vi "Read.vi"(8 "error in (no error)":errorcluster, 11 "Configuration Database API in":refnum<class "Configuration Database API.lvclass">) -> (0 "error out":errorcluster, 3 "Configuration Database API out":refnum<class "Configuration Database API.lvclass">)   [LabVIEW 2012, in "Configuration Database API.lvlib" / "Configuration Database API.lvclass"]
uses:
  Configuration Database API.lvclass
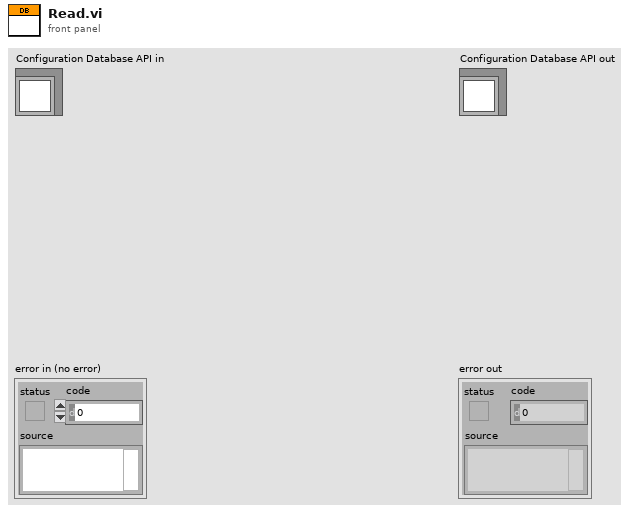
[diagram p1: front panel]
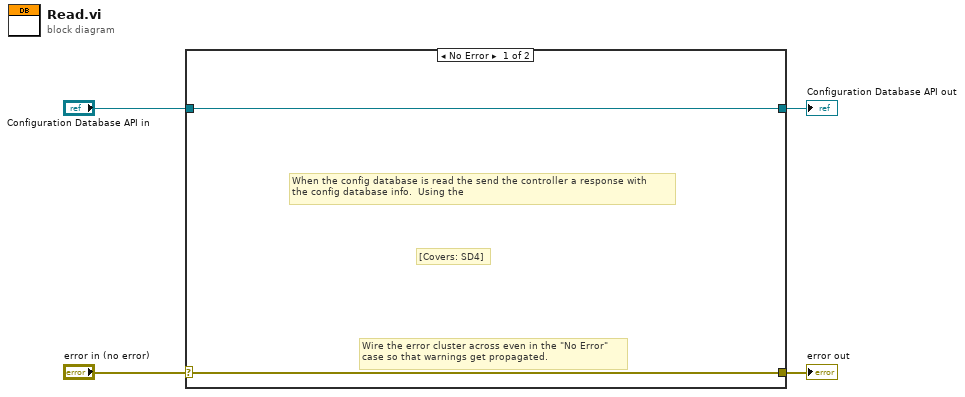
[diagram p0: block diagram]
diagram:
  n1 = case shown="No Error" "error in (no error)" {
    selector: "error in (no error)" -> [w5 w8]
    tunnel: [w5 w8] -> w3
    tunnel: [w6 w7] -> w1
    tunnel: "Configuration Database API in" -> [w6 w7]
    frame No Error {
      # "[Covers: SD4]"
      # "When the config database is read the send the controller a response with\nthe config database info.  Using the"
      # "Wire the error cluster across even in the \"No Error\"\ncase so that warnings get propagated."
    }
    frame Error {
    }
  }
  "error out" <- w3
  "Configuration Database API out" <- w1
